vi "Determine Analog and Digital Values for Channels.vi"(10 "Remaining Time":dbl, 11 "Step Settings":T1) -> (2 "Digital Values to Write":bool[](array[boolean]), 3 "Analog Values to Write":dbl[](array[numeric]))   [LabVIEW 2020, in "Sequencer with Output Values.lvlib" / "Sequencer with Output Values.lvclass"]
uses:
  Sequencer with Output Values.lvclass
  Step Settings.ctl
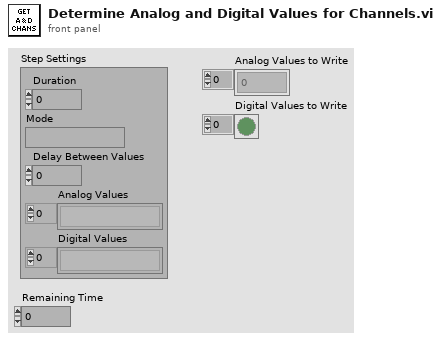
[diagram p1: front panel]
types:
  T1 = typedef "Sequencer with Output Values.lvlib/Sequencer with Output Values.lvclass/Step Settings.ctl" = cluster{"Duration":dbl, "Mode":string, "Delay Between Values":dbl, "Analog Values":string[], "Digital Values":string[]}
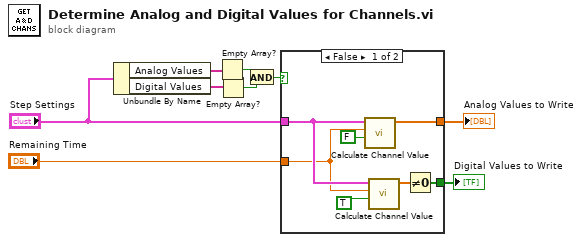
[diagram p0: block diagram]
diagram:
  n1 = Unbundle By Name("Step Settings") -> ("Analog Values"=w5:string[], "Digital Values"=w4:string[])
  n2 = Empty Array?(array=w5) -> (empty?=w3:bool)
  n3 = Empty Array?(array=w4) -> (empty?=w2:bool)
  n4 = And(x=w3, y=w2) -> (x .and. y?=w1:bool)
  n5 = case shown="False" w1 {
    tunnel: "Step Settings" -> [w15 _]
    tunnel: "Remaining Time" -> [w14 _]
    tunnel: [w12 _] -> w7
    tunnel: [w10 _] -> w6
    frame False {
      n6 = call "Calculate Channel Value.vi"("Digital"=FALSE, "Remaining Time"=w14, "Step Settings"=w15) -> ("Values to Write"=w12:dbl[])  [unwired: 8 in]
      n7 = call "Calculate Channel Value.vi"("Digital"=TRUE, "Remaining Time"=w14, "Step Settings"=w15) -> ("Values to Write"=w11:dbl[])  [unwired: 8 in]
      n8 = Not Equal To 0?(x=w11) -> (x != 0?=w10:bool[])
    }
    frame True {
      # "Don't need to worry about analog or digital channels if values arrays are empty"
    }
  }
  "Analog Values to Write" <- w7
  "Digital Values to Write" <- w6
